vi "Write f0.vi"(8 "error in (no error)":errorcluster, 10 "f0":i16, 11 "Send New Chirp MSG in":refnum<class "Send New Chirp MSG.lvclass">) -> (0 "error out":errorcluster, 3 "Send New Chirp MSG out":refnum<class "Send New Chirp MSG.lvclass">)   [LabVIEW 2014, in "ePAS Library.lvlib" / "Send New Chirp MSG.lvclass"]
uses:
  Send New Chirp MSG.lvclass
  Send New Chirp MSG.lvclass/Send New Chirp MSG.ctl
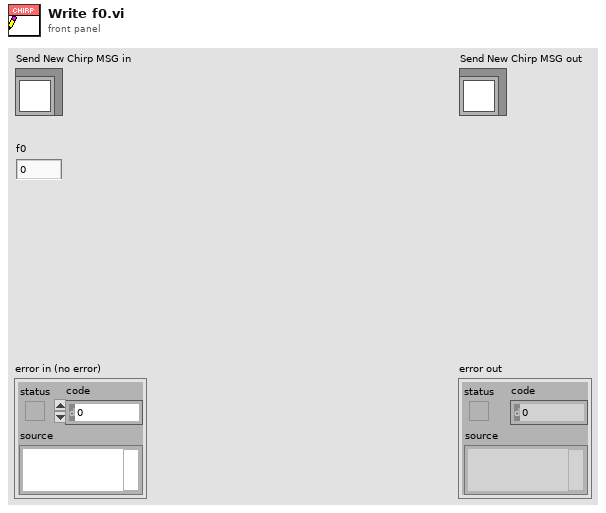
[diagram p1: front panel]
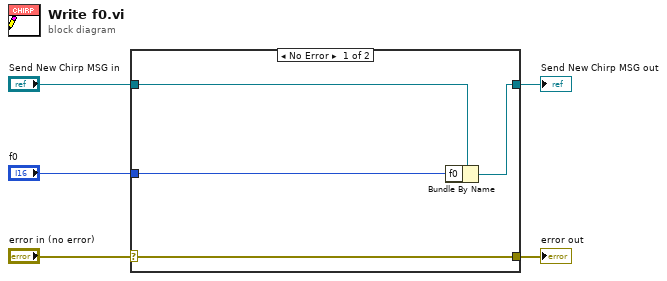
[diagram p0: block diagram]
diagram:
  n1 = case shown="No Error" "error in (no error)" {
    selector: "error in (no error)" -> [w9 w10]
    tunnel: [w9 w10] -> w4
    tunnel: [w7 w11] -> w2
    tunnel: "Send New Chirp MSG in" -> [w8 w11]
    tunnel: "f0" -> [w6 _]
    frame No Error {
      n2 = Bundle By Name(cluster=w8, "f0"=w6) -> (w7:refnum<class "Send New Chirp MSG.lvclass">)
    }
    frame Error {
    }
  }
  "error out" <- w4
  "Send New Chirp MSG out" <- w2
